vi "Conditional Concatenating of String Array.vi"(0 "Array In":string[](array[string]), 1 "New Items":string[](array[string]), 9 "Concatenate?":bool) -> (14 "Array Out":string[](array[string]))   [LabVIEW 2014]
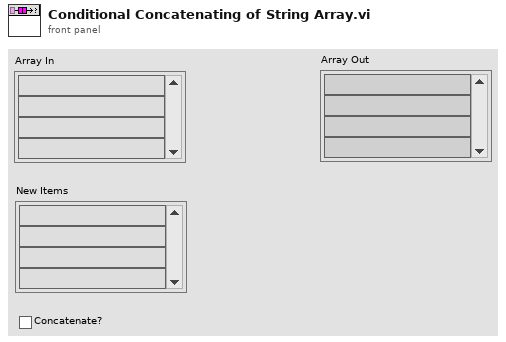
[diagram p1: front panel]
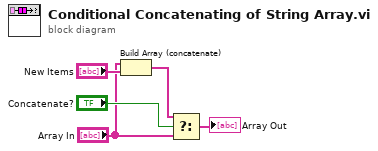
[diagram p0: block diagram]
diagram:
  n1 = Build Array (concatenate)("Array In", "New Items") -> (w3:string[])
  n2 = Select(t=w3, s="Concatenate?", f="Array In") -> (s? t:f=→"Array Out":string[])
